vi "Handshake.vi"(8 "error in (no error)":errorcluster, 9 "Timeout (5000ms)":u32=5000, 11 "OpenSSL in":refnum<class "SSL Socket.lvclass">) -> (0 "error out":errorcluster, 3 "OpenSSL out":refnum<class "SSL Socket.lvclass">)   [LabVIEW 2013, in "OpenSSL Socket.lvlib" / "SSL Socket.lvclass"]
uses:
  SSL Socket.lvclass
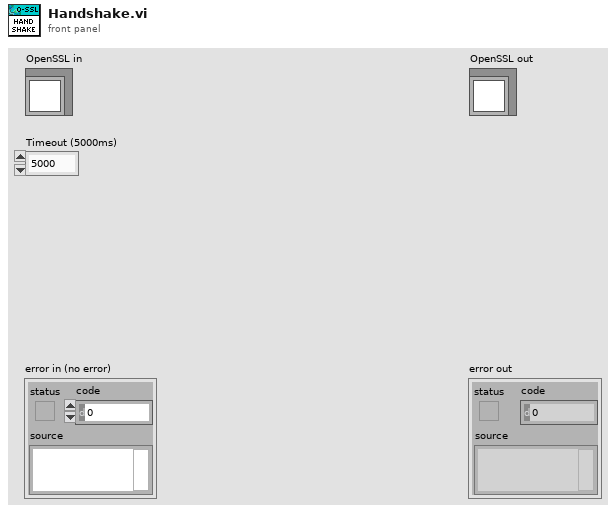
[diagram p1: front panel]
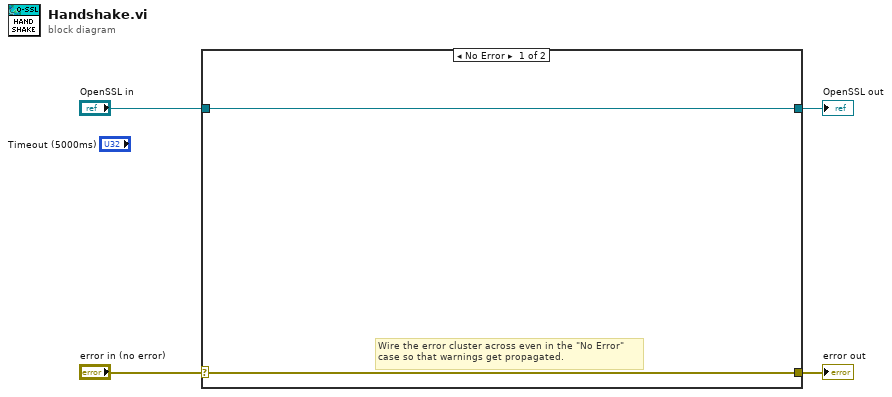
[diagram p0: block diagram]
diagram:
  n1 = case shown="No Error" "error in (no error)" {
    selector: "error in (no error)" -> [w5 w8]
    tunnel: [w5 w8] -> w3
    tunnel: [w6 w7] -> w1
    tunnel: "OpenSSL in" -> [w6 w7]
    frame No Error {
      # "Wire the error cluster across even in the \"No Error\"\ncase so that warnings get propagated."
    }
    frame Error {
    }
  }
  "error out" <- w3
  "OpenSSL out" <- w1
